vi "CuLab_Windowing_CSG.vi"(7 "window":u16(ring) items=["None "=0, "Hanning"=1, "Hamming"=2, "Blackman-Harris"=3, "Exact Blackman"=4, "Blackman"=5, "Flat Top"=6, "4 Term B-Harris "=7, "7 Term B-Harris"=8, "Low Sidelobe"=9, "Blackman Nuttall"=11], 8 "error in (no error)":errorcluster, 11 "T1D_CSG in":refnum<class "T1D_CSG.lvclass">) -> (0 "error out":errorcluster, 3 "T1D_CSG out":refnum<class "T1D_CSG.lvclass">)   [LabVIEW 2020]
uses:
  <vilib>/Ngene/CuLab - GPU Accelerated Toolkit/Toolkit/Low_Level/Tensor_Classes/T_Children/T1D/T1D_Children/T1D_CSG/T1D_CSG.lvclass
  C:/Program Files/National Instruments/LabVIEW 2020/vi.lib/Ngene/CuLab - GPU Accelerated Toolkit/Toolkit/Low_Level/Tensor_Classes/T_Children/T1D/T1D.lvclass
  C:/Program Files/National Instruments/LabVIEW 2020/vi.lib/Ngene/CuLab - GPU Accelerated Toolkit/Toolkit/Low_Level/Tensor_Classes/Tensor.lvclass
  93686d1c-d6de-4b16-a0fc-7f36ed8a1a68.vi
  0b8842e4-a500-4db8-ba12-85dbe126322b.vi
  <vilib>/Ngene/CuLab - GPU Accelerated Toolkit/Toolkit/API/Array/Array Size/CU_Array_Size_T1D.vi
  <vilib>/Ngene/CuLab - GPU Accelerated Toolkit/Toolkit/Low_Level/Tensor_Classes/T_Children/T1D/T1D_Children/T1D_CSG/Create_Push.vi
  <vilib>/Ngene/CuLab - GPU Accelerated Toolkit/Toolkit/API/Numeric/Multiply/T1D/CU_Multiply_T1D_CSG.vi
  <vilib>/Ngene/CuLab - GPU Accelerated Toolkit/Toolkit/CuLab.lvlib
  <vilib>/Analysis/NI_AALPro.lvlib
  C:/Program Files/National Instruments/LabVIEW 2020/vi.lib/Ngene/CuLab - GPU Accelerated Toolkit/Toolkit/Low_Level/Tensor_Classes/T_Children/T1D/T1D_Children/T1D_CSG/T1D_CSG.lvclass
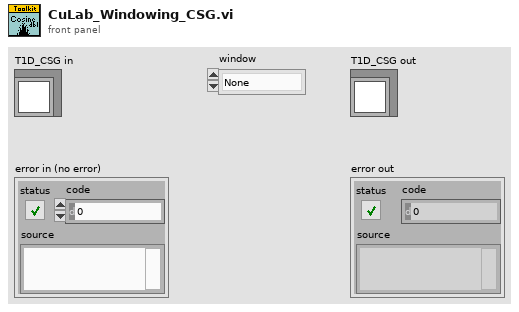
[diagram p1: front panel]
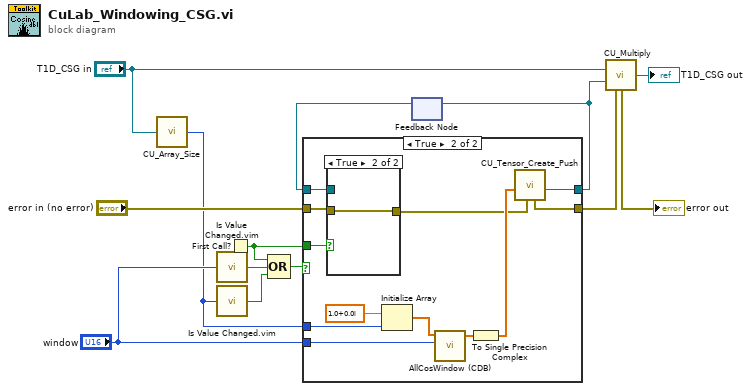
[diagram p0: block diagram]
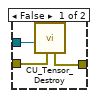
[diagram p3: hidden frame]
diagram:
  n1 = call-poly <vilib>:"CU_Array_Size.vi"("Tensor"="T1D_CSG in") -> ("size"=w5:i32)  [unwired: 14 in]
  n2 = call "Is Value Changed.vim"("value"="window") -> ("changed or first call?"=w8:bool)
  n3 = call "Is Value Changed.vim"("value"=w5) -> ("changed or first call?"=w4:bool)
  n4 = First Call?() -> (First Call?: T/F=w7:bool)
  n5 = Compound Arithmetic op=OR(w7, w8, w4) -> (w6:bool)
  n6 = feedback #1() -> (w13:refnum<class "T1D_CSG.lvclass">)  [unwired: 1 in]
  n7 = case shown="True" w6 {
    tunnel: w13 -> [w15 w27]
    tunnel: "error in (no error)" -> [w14 w26]
    tunnel: "window" -> [_ w25]
    tunnel: [w14 w16] -> w9
    tunnel: w7 -> [_ w24]
    tunnel: [w15 w22] -> w1
    tunnel: w5 -> [_ w20]
    frame False {
    }
    frame True {
      n8 = case shown="True" w24 {
        tunnel: w27 -> [w30 _]
        tunnel: w26 -> [w29 w31]
        tunnel: [w28 w31] -> w17
        frame False {
          n9 = call <vilib>:"CU_Tensor_Destroy.vi"("error in (no error)"=w29, "Tensor in"=w30) -> ("error out"=w28:errorcluster)  [unwired: 9 in]
        }
        frame True {
        }
      }
      n10 = Initialize Array(cdb 1.0+0.0i ("element"), w20) -> (w18:cdb[])
      n11 = call <vilib>:"AllCosWindow (CDB).vi"("window"=w25, "X"=w18) -> ("Windowed X"=w23:cdb[])  [unwired: 3 in, 1 out]
      n12 = To Single Precision Complex(1:w23) -> (0:w21:csg[])
      n13 = call-poly <vilib>:"CU_Tensor_Create_Push.vi"("error in (no error)"=w17, "CPU_Data_1D_CSG"=w21) -> ("T1D_CSG out"=w22:refnum<class "T1D_CSG.lvclass">, "error out"=w16:errorcluster)  [unwired: 8 in]
    }
  }
  n14 = feedback-in #1(w1) -> ()
  n15 = call-poly <vilib>:"CU_Multiply.vi"("x"="T1D_CSG in", "y"=w1, "error in (no error)"=w9) -> ("Dest out"=→"T1D_CSG out":refnum<class "T1D_CSG.lvclass">, "error out"=→"error out":errorcluster)  [unwired: 11 in]
